vi "Single Measure Reference.vi"(7 "High Reference":dbl, 8 "error in":errorcluster, 9 "Mid Reference":dbl, 10 "Low Reference":dbl, 11 "Instrument Handle In":i32) -> (0 "error out":errorcluster, 3 "Instrument Handle Out":i32)   [LabVIEW 8.6, in "ZTScopeM.lvlib"]
doc: "Configure the voltage threshold levels for measurements.\nValues may be in either volts or percent depending on the reference method. By default, the low level is 10% of the waveform, the mid level is 50%, and the high level is 90%."
uses:
  ZTScopeM.lvlib
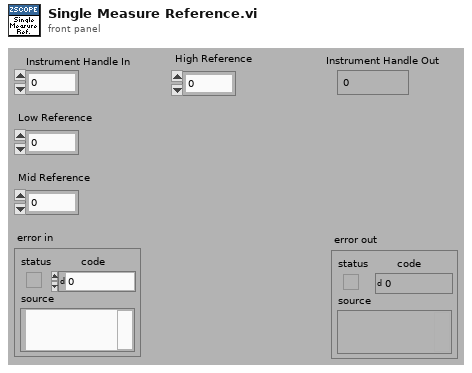
[diagram p1: front panel]
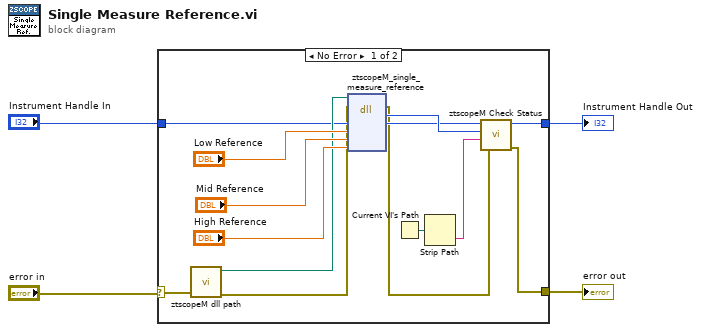
[diagram p0: block diagram]
diagram:
  n1 = case shown="No Error" "error in" {
    selector: "error in" -> [w9 w20]
    tunnel: [w13 w20] -> w3
    tunnel: [w14 w19] -> w2
    tunnel: "Instrument Handle In" -> [w7 w19]
    frame #0 {
      n2 = call "ztscopeM dll path.vi"("error in (no error)"=w9) -> ("error out"=w6:errorcluster, "<instrument>.dll path"=w8:path)  [unwired: 9 in]
      n3 = dll-call lib="C:/Program Files (x86)/National Instruments/LabVIEW 2013/instr.lib/ztscopem/ztscopeM.dll" fn="ztscopeM_single_measure_reference"(path in=w8, error in=w6, "instrumentHandle"=w7, "lowReference"="Low Reference", "midReference"="Mid Reference", "highReference"="High Reference") -> (error out=w5:errorcluster, w18:i32, "instrumentHandle"=w17:i32)  [unwired: 4 in, 1 out]
      n4 = Current VI's Path() -> (path=w16:path)
      n5 = Strip Path(path=w16) -> (name=w15:string)  [unwired: 1 out]
      n6 = call "ztscopeM Check Status.vi"("error in"=w5, "name of VI"=w15, "status (return code)"=w18, "instrument handle in"=w17) -> ("error out"=w13:errorcluster, "instrument handle out"=w14:i32)  [unwired: 2 out]
    }
    frame #1 {
    }
  }
  "Instrument Handle Out" <- w2
  "error out" <- w3
